vi "Calculate_Linearity_Persentage_of_Subtrack-1.vi"(6 "[IN] Max angle":dbl, 7 "[IN] Subtrack":T1) -> (3 "[OUT] Track Linearity in %":u8)   [LabVIEW 2013]
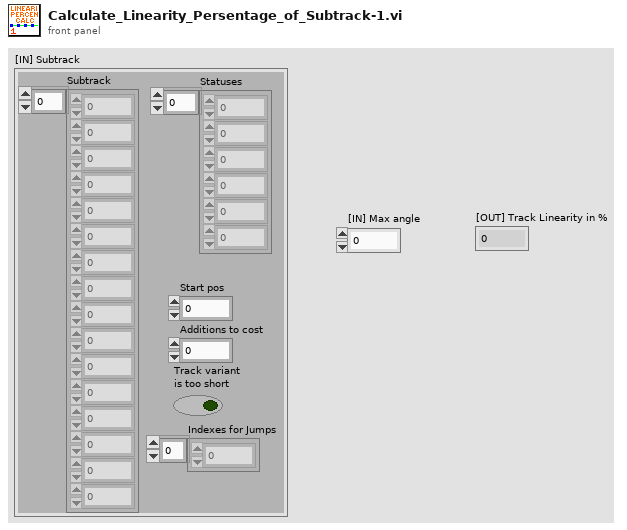
[diagram p1: front panel]
types:
  T1 = cluster{"Subtrack":dbl[], "Statuses":i16[], "Start pos":i32, "Additions to cost":i8, "Track variant \nis too short":bool, "Indexes for Jumps":i32[]}
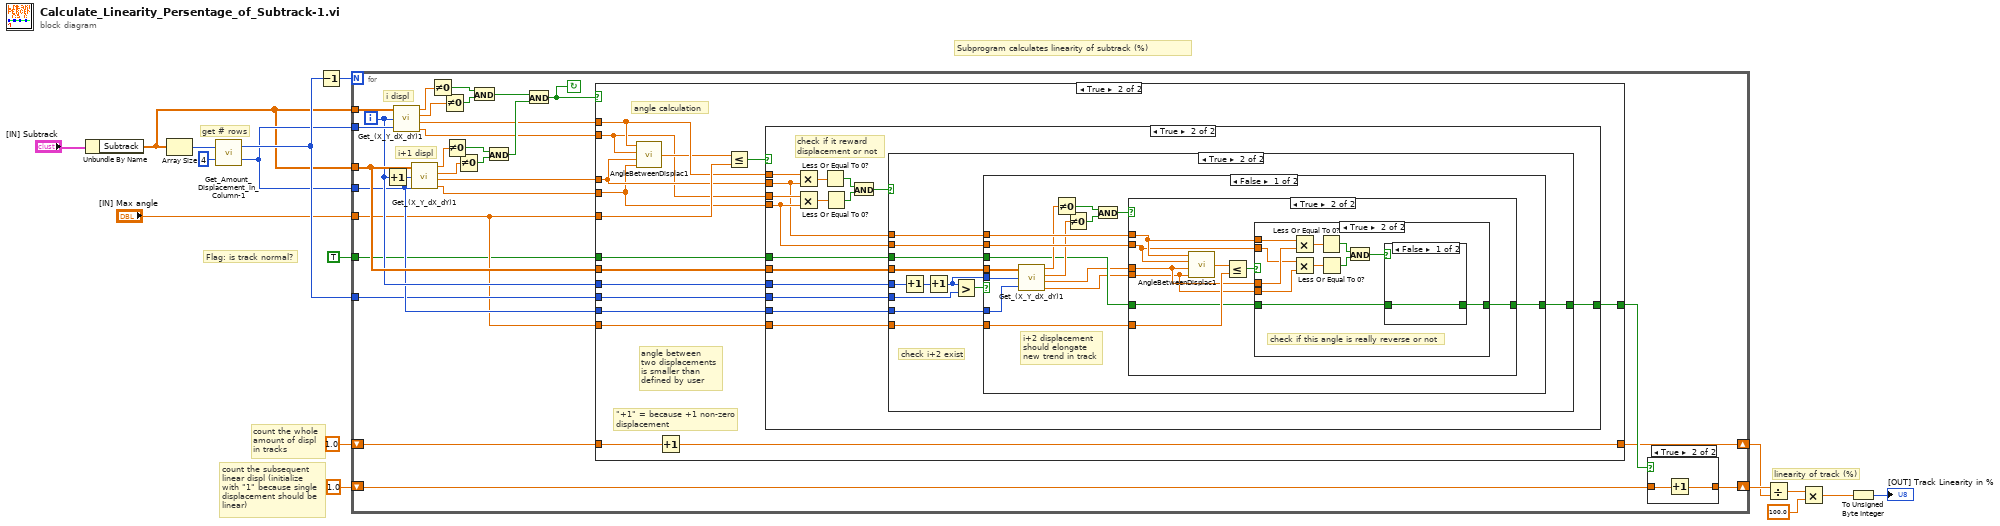
[diagram p0: block diagram]
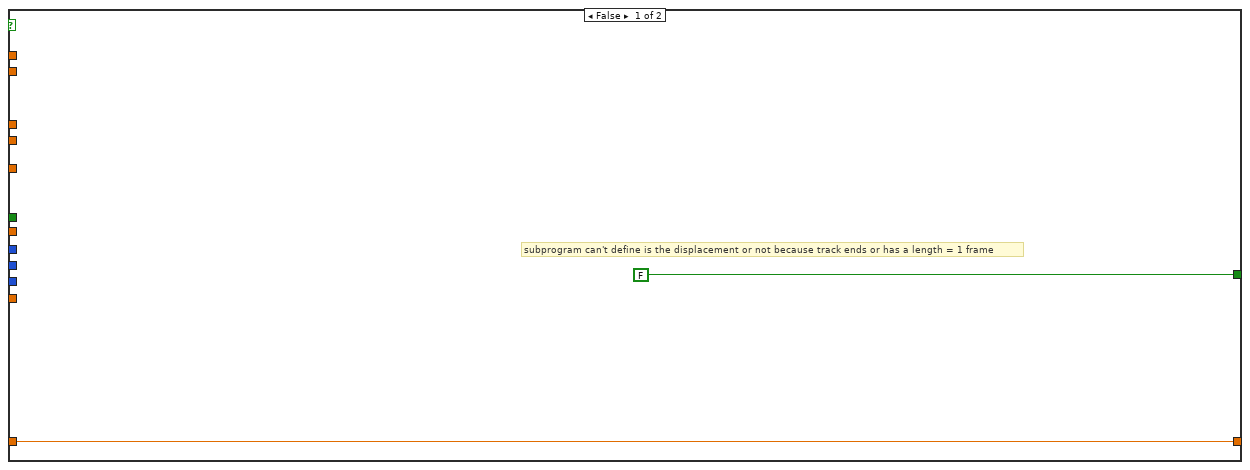
[diagram p3: hidden frame]
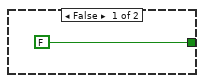
[diagram p4: hidden frame]
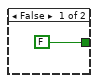
[diagram p6: hidden frame]
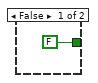
[diagram p7: hidden frame]
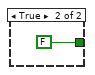
[diagram p8: hidden frame]
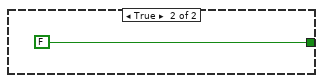
[diagram p9: hidden frame]
diagram:
  # "Subprogram calculates linearity of subtrack (%)"
  # "get # rows"
  # "linearity of track (%)"
  # "count the subsequent\nlinear displ (initialize \nwith \"1\" because single\ndisplacement should be\nlinear)"
  # "count the whole\namount of displ\nin tracks"
  # "Flag: is track normal?"
  n1 = Unbundle By Name("[IN] Subtrack") -> ("Subtrack"=w4:dbl[])
  n2 = Array Size(array=w4) -> (size(s)=w8:i32)
  n3 = call "Get_Amount_Displacement_in_Column-1.vi"("multiplier"=4, "# Rows"=w8) -> ("multiplier out"=w6:i32, "Displ amount"=w7:i32)
  n4 = Decrement(x=w7) -> (x-1=w17:i32)
  n5 = for {
    N: w17 -> [_]
    tunnel: w4 -> [w46]
    tunnel: w6 -> [w40]
    tunnel: w4 -> [w32]
    tunnel: w6 -> [w30]
    tunnel: "[IN] Max angle" -> [w25]
    tunnel: w7 -> [w26]
    tunnel: TRUE -> [w24]
    shift-right: [w20] -> w12
    shift-left: 1.0 -> [w21]
    shift-right: [w18] -> w13
    shift-left: 1.0 -> [w19]
    i -> [w31]
    stop <- w23 continue-if-true
    # "i+1 displ"
    # "i displ"
    n6 = Increment(x=w31) -> (x+1=w41:i32)
    n7 = call "Get_(X_Y_dX_dY)1.vi"("(X,Y,dX,dY)"=w46, "index"=w31, "multiplier"=w40) -> ("X"=w45:dbl, "Y"=w44:dbl, "dX"=w29:dbl, "dY"=w33:dbl)
    n8 = call "Get_(X_Y_dX_dY)1.vi"("(X,Y,dX,dY)"=w32, "index"=w41, "multiplier"=w30) -> ("X"=w37:dbl, "Y"=w36:dbl, "dX"=w28:dbl, "dY"=w27:dbl)
    n9 = Not Equal To 0?(x=w45) -> (x != 0?=w42:bool)
    n10 = Not Equal To 0?(x=w44) -> (x != 0?=w43:bool)
    n11 = Not Equal To 0?(x=w37) -> (x != 0?=w38:bool)
    n12 = Not Equal To 0?(x=w36) -> (x != 0?=w39:bool)
    n13 = And(x=w42, y=w43) -> (x .and. y?=w35:bool)
    n14 = And(x=w38, y=w39) -> (x .and. y?=w34:bool)
    n15 = And(x=w35, y=w34) -> (x .and. y?=w23:bool)
    n16 = case shown="True" w23 {
      tunnel: w33 -> [_ w57]
      tunnel: w29 -> [_ w60]
      tunnel: w28 -> [_ w58]
      tunnel: w27 -> [_ w56]
      tunnel: w25 -> [_ w67]
      tunnel: w24 -> [_ w65]
      tunnel: [FALSE w64] -> w22
      tunnel: w32 -> [_ w63]
      tunnel: w31 -> [_ w62]
      tunnel: w30 -> [_ w61]
      tunnel: w26 -> [_ w55]
      tunnel: w25 -> [_ w54]
      tunnel: w21 -> [w51 w52]
      tunnel: [w51 w53] -> w20
      frame False {
        # "subprogram can't define is the displacement or not because track ends or has a length = 1 frame"
      }
      frame True {
        # "\"+1\" = because +1 non-zero\ndisplacement"
        # "angle calculation"
        # "angle between\ntwo displacements\nis smaller than \ndefined by user"
        n17 = call "AngleBetweenDisplac1.vi"("dY 2"=w56, "dX 2"=w58, "dY 1"=w57, "dX 1"=w60) -> ("angle in degrees"=w59:dbl)
        n18 = Increment(x=w52) -> (x+1=w53:dbl)
        n19 = Less Or Equal?(x=w59, y=w67) -> (x <= y?=w66:bool)
        n20 = case shown="True" w66 {
          tunnel: w58 -> [_ w69]
          tunnel: w56 -> [_ w71]
          tunnel: w60 -> [_ w84]
          tunnel: w57 -> [_ w72]
          tunnel: w65 -> [_ w78]
          tunnel: [FALSE w77] -> w64
          tunnel: w63 -> [_ w76]
          tunnel: w62 -> [_ w75]
          tunnel: w61 -> [_ w74]
          tunnel: w55 -> [_ w73]
          tunnel: w54 -> [_ w70]
          frame False {
          }
          frame True {
            # "check if it reward \ndisplacement or not"
            n21 = Multiply(x=w84, y=w69) -> (x*y=w83:dbl)
            n22 = Multiply(x=w72, y=w71) -> (x*y=w82:dbl)
            n23 = Less Or Equal To 0?(x=w83) -> (x <= 0?=w80:bool)
            n24 = Less Or Equal To 0?(x=w82) -> (x <= 0?=w81:bool)
            n25 = And(x=w80, y=w81) -> (x .and. y?=w79:bool)
            n26 = case shown="True" w79 {
              tunnel: w78 -> [w85 w93]
              tunnel: [w85 w92] -> w77
              tunnel: w76 -> [_ w91]
              tunnel: w75 -> [_ w97]
              tunnel: w74 -> [_ w89]
              tunnel: w73 -> [_ w95]
              tunnel: w69 -> [_ w88]
              tunnel: w71 -> [_ w87]
              tunnel: w70 -> [_ w86]
              frame False {
              }
              frame True {
                # "check i+2 exist"
                n27 = Increment(x=w97) -> (x+1=w96:i32)
                n28 = Increment(x=w96) -> (x+1=w90:i32)
                n29 = Greater?(x=w90, y=w95) -> (0:w94:bool)
                n30 = case shown="False" w94 {
                  tunnel: w93 -> [w102 _]
                  tunnel: [w98 FALSE] -> w92
                  tunnel: w91 -> [w109 _]
                  tunnel: w90 -> [w108 _]
                  tunnel: w89 -> [w107 _]
                  tunnel: w88 -> [w106 _]
                  tunnel: w87 -> [w105 _]
                  tunnel: w86 -> [w101 _]
                  frame False {
                    # "i+2 displacement \nshould elongate\nnew trend in track"
                    n31 = call "Get_(X_Y_dX_dY)1.vi"("(X,Y,dX,dY)"=w109, "index"=w108, "multiplier"=w107) -> ("X"=w104:dbl, "Y"=w103:dbl, "dX"=w100:dbl, "dY"=w99:dbl)
                    n32 = Not Equal To 0?(x=w104) -> (x != 0?=w112:bool)
                    n33 = Not Equal To 0?(x=w103) -> (x != 0?=w111:bool)
                    n34 = And(x=w112, y=w111) -> (x .and. y?=w110:bool)
                    n35 = case shown="True" w110 {
                      tunnel: [FALSE w114] -> w98
                      tunnel: w106 -> [_ w119]
                      tunnel: w105 -> [_ w116]
                      tunnel: w100 -> [_ w118]
                      tunnel: w99 -> [_ w117]
                      tunnel: w102 -> [_ w115]
                      tunnel: w101 -> [_ w121]
                      frame False {
                      }
                      frame True {
                        n36 = call "AngleBetweenDisplac1.vi"("dY 2"=w117, "dX 2"=w118, "dY 1"=w116, "dX 1"=w119) -> ("angle in degrees"=w122:dbl)
                        n37 = Less Or Equal?(x=w122, y=w121) -> (x <= y?=w120:bool)
                        n38 = case shown="True" w120 {
                          tunnel: w119 -> [_ w130]
                          tunnel: w118 -> [_ w129]
                          tunnel: w117 -> [_ w128]
                          tunnel: w116 -> [_ w127]
                          tunnel: w115 -> [_ w125]
                          tunnel: [FALSE w124] -> w114
                          frame False {
                          }
                          frame True {
                            # "check if this angle is really reverse or not"
                            n39 = Multiply(x=w130, y=w129) -> (x*y=w134:dbl)
                            n40 = Multiply(x=w127, y=w128) -> (x*y=w133:dbl)
                            n41 = Less Or Equal To 0?(x=w134) -> (x <= 0?=w131:bool)
                            n42 = Less Or Equal To 0?(x=w133) -> (x <= 0?=w132:bool)
                            n43 = And(x=w131, y=w132) -> (x .and. y?=w126:bool)
                            n44 = case shown="False" w126 {
                              tunnel: w125 -> [w135 _]
                              tunnel: [w135 FALSE] -> w124
                              frame False {
                              }
                              frame True {
                              }
                            }
                          }
                        }
                      }
                    }
                  }
                  frame True {
                  }
                }
              }
            }
          }
        }
      }
    }
    n45 = case shown="True" w22 {
      tunnel: w19 -> [w47 w49]
      tunnel: [w47 w48] -> w18
      frame False {
      }
      frame True {
        n46 = Increment(x=w49) -> (x+1=w48:dbl)
      }
    }
  }
  n47 = Divide(x=w13, y=w12) -> (x/y=w11:dbl)
  n48 = Multiply(x=w11, y=100.0) -> (x*y=w2:dbl)
  n49 = To Unsigned Byte Integer(number=w2) -> (unsigned 8bit integer=→"[OUT] Track Linearity in %":u8)
